vi "_Clear Listbox - FP.vi"(0 "GObject in":refnum<vi>, 5 "error in (no error)":errorcluster) -> (14 "changed?":bool, 19 "error out":errorcluster)   [LabVIEW 2017, in "QD_Erease Data.lvlib"]
uses:
  QD_Erease Data.lvlib
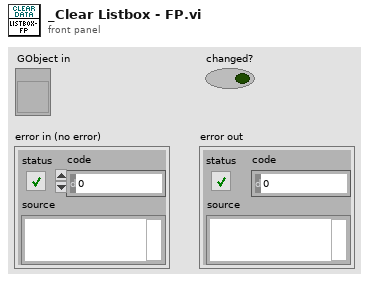
[diagram p1: front panel]
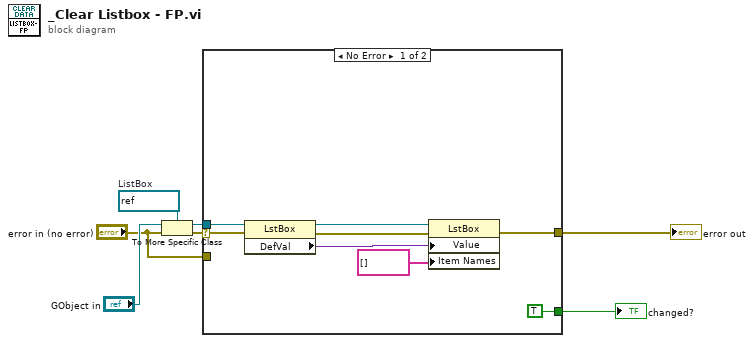
[diagram p0: block diagram]
diagram:
  w6 = refnum<vi> refnum  # ListBox
  n1 = To More Specific Class(target class=w6, reference="GObject in", error in="error in (no error)") -> (specific class reference=w2:refnum<vi>, error out=w3:errorcluster)
  n2 = case shown="No Error" w3 {
    selector: w3 -> [w10 _]
    tunnel: [w15 w16] -> w1
    tunnel: w2 -> [w13 _]
    tunnel: "error in (no error)" -> [_ w16]
    tunnel: [TRUE _] -> w7
    frame No Error {
      n3 = property class="LstBox"(reference=w13, error in=w10) -> (reference out=w11:refnum<vi>, error out=w9:errorcluster, "DefVal"=w8:variant)
      n4 = property class="LstBox"(reference=w11, error in=w9, "Value"=w8, "Item Names"=string[] []) -> (error out=w15:errorcluster)  [unwired: 1 out]
    }
    frame Error {
    }
  }
  "changed?" <- w7
  "error out" <- w1
